vi "MinMax_getInfo.vi"(6 "error in (no error)":errorcluster, 7 "Current Channel":string, 8 "Node Path Array":string[](array[string]), 9 "Ref In":T1) -> (0 "error out":errorcluster, 1 "System Time":dbl, 2 "Current Value":dbl, 3 "Ref Out":T1)   [LabVIEW 2010]
uses:
  <vilib>/NI Veristand/Execution/Workspace/WorkspaceAPI.ctl
  NationalInstruments.VeriStand.ClientAPI
  <vilib>/NI VeriStand/Execution/Workspace/NI VeriStand - Get Multiple Channel Values.vi
  <vilib>/NI Veristand/Execution/Workspace/NI_VS Workspace ExecutionAPI.lvlib
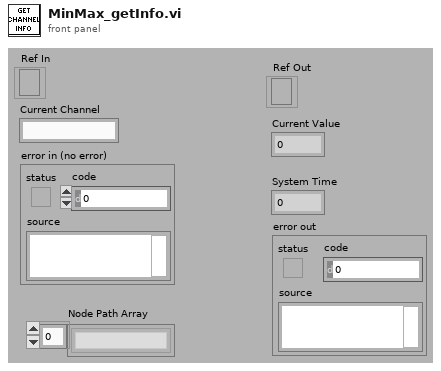
[diagram p1: front panel]
types:
  T1 = typedef "NI_VS Workspace ExecutionAPI.lvlib/WorkspaceAPI.ctl" = refnum<k24>
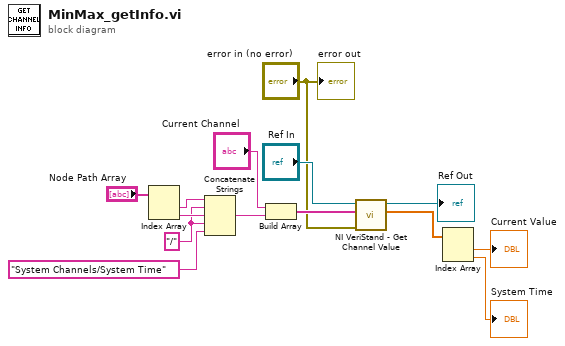
[diagram p0: block diagram]
diagram:
  w3 = "/" ("Channel")
  n1 = Index Array(array="Node Path Array") -> (element #1=w5:string, element #2=w4:string)  [unwired: 2 in]
  n2 = Concatenate Strings(w5, w3, w4, w3, "System Channels/System Time" ("string")) -> (w1:string)
  n3 = Build Array("Current Channel", w1) -> (w11:string[])
  n4 = call-poly <vilib>:"NI VeriStand - Get Channel Value.vi"("error in (no error)"="error in (no error)", "Channels"=w11, "WorkspaceManager in"="Ref In") -> ("Values"=w12:dbl[], "WorkspaceManager out"=→"Ref Out":T1)  [unwired: 6 in, 1 out]
  n5 = Index Array(array=w12) -> (element #1=→"Current Value":dbl, element #2=→"System Time":dbl)  [unwired: 2 in]
  "error out" <- "error in (no error)"
